vi "Terminal_Global_Alarm_condition.vi"() -> ()   [LabVIEW 2014]
panel:
  in  "监测量报警条件":string[][](table)
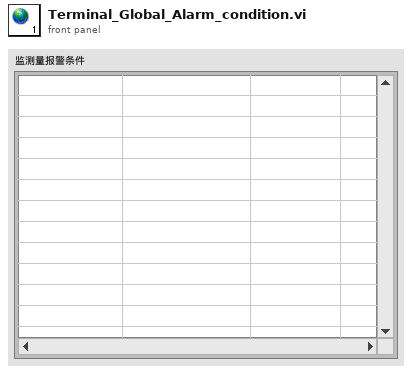
[diagram p1: front panel]
diagram:
